vi "150327-Counter-FiniteOutput.vi"(8 "error in":errorcluster, 9 "Number of Pulses":i32=1800, 10 "Frequency":dbl=10.0 format="%.6f") -> (0 "error out 2":errorcluster)   [LabVIEW 2013]
doc: "This example demonstrates how to generate a finite number of digital pulses using a counter output.\n\nOn some hardware, this requires the use of a second counter to generate a gate signal. If necessary, DAQmx configures this second counter for you."
uses:
  <vilib>/Utility/error.llb/DialogType.ctl
  <vilib>/DAQmx/create/channels.llb/DAQmx Create Channel (CO-Pulse Generation-Frequency).vi
  <vilib>/DAQmx/configure/timing.llb/DAQmx Timing (Implicit).vi
  <vilib>/DAQmx/configure/trigger.llb/DAQmx Start Trigger (Digital Edge).vi
  <resource>/objmgr/daqmx.rc
panel:
  out "Actual Duty Cycle":dbl=0.5
  out "Actual Frequency":dbl=10.0
  in  "Duty Cycle":dbl=0.5 format="%.6f"
  in  "Output Terminal":tag="/Dev4/PFI24"
  in  "Trigger Type":enum32{"No Trigger", "Digital Start"}(tab)
  in  "Retriggerable":bool
  in  "Edge":i32(ring)=10280 items=["Rising"=10280, "Falling"=10171]
  in  "Digital Trigger Source":tag
  in  "Stop":bool
  in  "Counter":tag="Dev4/ctr3"
  # "Channel Settings"
  # "Timing Settings"
  # "Trigger Settings"
  # "To configure and use a trigger you must have the necessary tab selected above."
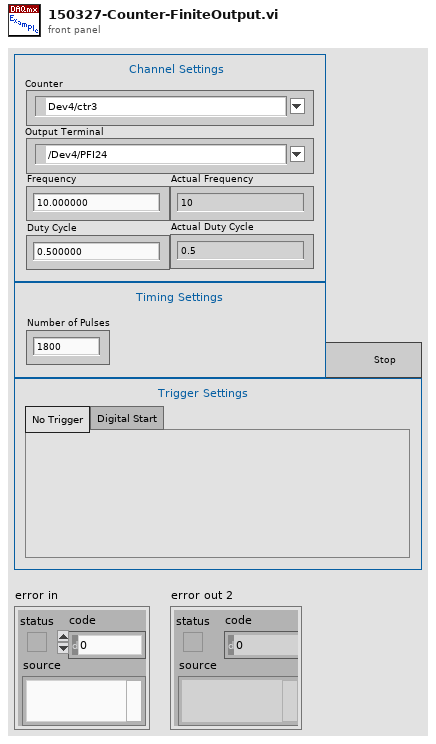
[diagram p1: front panel]
types:
  T1 = typedef "DialogType.ctl" = u16
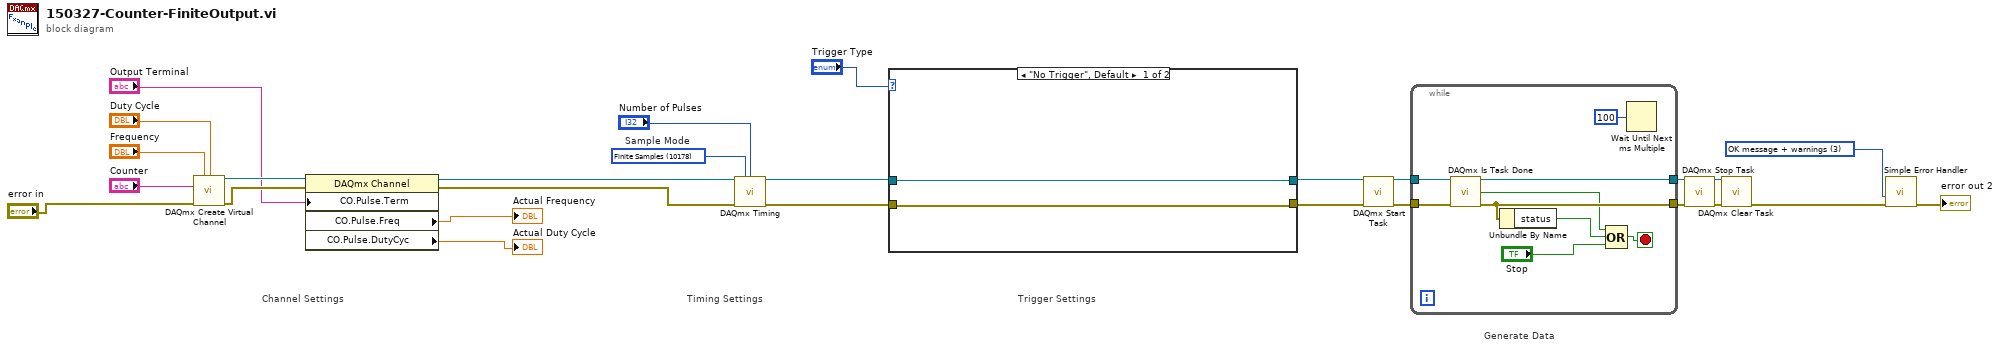
[diagram p0: block diagram]
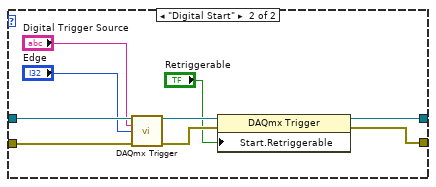
[diagram p2: hidden frame]
diagram:
  w3 = T1 3 items=["no dialog", "OK message", "continue or stop message", "OK message + warnings", "continue/stop + warnings"] ("type of dialog (OK msg:1)")
  w27 = 10178 items=["Finite Samples"=10178, "Continuous Samples"=10123, "Hardware Timed Single Point"=12522]  # Sample Mode
  # "Generate Data"
  # "Trigger Settings"
  # "Timing Settings"
  # "Channel Settings"
  n1 = call-poly <vilib>:"DAQmx Create Virtual Channel.vi"("frequency"="Frequency", "duty cycle"="Duty Cycle", "counter"="Counter", "error in"="error in") -> ("task out"=w17:refnum<k21>, "error out"=w16:errorcluster)  [unwired: 10 in]
  n2 = property class="DAQmx Channel"(reference=w17, error in=w16, "CO.Pulse.Term"="Output Terminal") -> (reference out=w13:refnum<k21>, error out=w14:errorcluster, "CO.Pulse.Freq"=→"Actual Frequency":dbl, "CO.Pulse.DutyCyc"=→"Actual Duty Cycle":dbl)
  n3 = call-poly <vilib>:"DAQmx Timing.vi"("task/channels in"=w13, "sample mode"=w27, "samples per channel"="Number of Pulses", "error in"=w14) -> ("task out"=w21:refnum<k21>, "error out"=w20:errorcluster)  [unwired: 10 in]
  n4 = case shown="\"No Trigger\", Default" "Trigger Type" {
    tunnel: w21 -> [w29 w38]
    tunnel: w20 -> [w28 w37]
    tunnel: [w29 w34] -> w18
    tunnel: [w28 w33] -> w19
    frame "No Trigger", Default {
    }
    frame "Digital Start" {
      n5 = call-poly <vilib>:"DAQmx Trigger.vi"("task/channels in"=w38, "source"="Digital Trigger Source", "edge"="Edge", "error in"=w37) -> ("task out"=w31:refnum<k21>, "error out"=w32:errorcluster)  [unwired: 10 in]
      n6 = property class="DAQmx Trigger"(reference=w31, error in=w32, "Start.Retriggerable"="Retriggerable") -> (reference out=w34:refnum<k21>, error out=w33:errorcluster)
    }
  }
  n7 = call <vilib>:"DAQmx Start Task.vi"("task/channels in"=w18, "error in"=w19) -> ("task out"=w26:refnum<k21>, "error out"=w25:errorcluster)  [unwired: 12 in]
  n8 = while {
    tunnel: w26 -> [w47]
    tunnel: w25 -> [w46]
    tunnel: [w43] -> w4
    tunnel: [w44] -> w5
    stop <- w45 stop-if-true
    n9 = call <vilib>:"DAQmx Is Task Done.vi"("task/channels in"=w47, "error in"=w46) -> ("task out"=w44:refnum<k21>, "task done?"=w40:bool, "error out"=w43:errorcluster)  [unwired: 11 in]
    n10 = Unbundle By Name(w43) -> ("status"=w42:bool)
    n11 = Compound Arithmetic op=OR(w40, w42, "Stop") -> (w45:bool)
    n12 = Wait Until Next ms Multiple(millisecond multiple=u32 100) -> ()  [unwired: 1 out]
  }
  n13 = call <vilib>:"DAQmx Stop Task.vi"("task/channels in"=w5, "error in"=w4) -> ("task out"=w7:refnum<k21>, "error out"=w6:errorcluster)  [unwired: 12 in]
  n14 = call <vilib>:"DAQmx Clear Task.vi"("task in"=w7, "error in"=w6) -> ("error out"=w24:errorcluster)  [unwired: 13 in]
  n15 = call <vilib>:"Simple Error Handler.vi"("type of dialog (OK msg:1)"=w3, "error in (no error)"=w24) -> ("error out"=→"error out 2":errorcluster)  [unwired: 3 in, 4 out]
